vi "Variant_to_String.vi"(3 "error in (no error)":errorcluster, 5 "Variant":variant) -> (0 "error out":errorcluster, 2 "String":string)   [LabVIEW 2015]
doc: "Use this VI to change any data into a string."
panel:
  # "Creator: Branson Darnell\nEmail: bdarnell@enviroptics.com\n\nEmail me if you encounter issues with this VI."
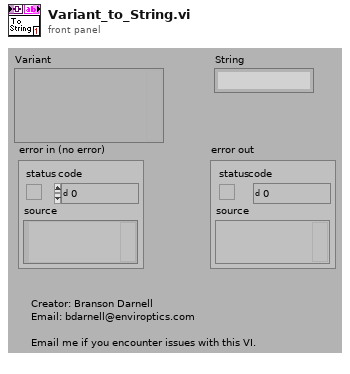
[diagram p1: front panel]
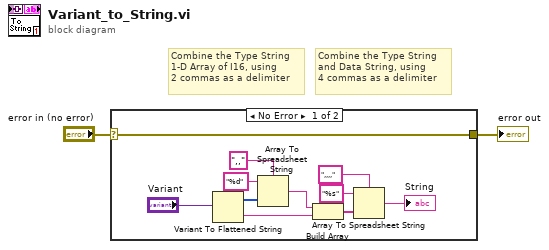
[diagram p0: block diagram]
diagram:
  # "Combine the Type String\nand Data String, using\n4 commas as a delimiter"
  # "Combine the Type String\n1-D Array of I16, using\n2 commas as a delimiter"
  n1 = case shown="No Error" "error in (no error)" {
    selector: "error in (no error)" -> [w7 w14]
    tunnel: [w7 w14] -> w1
    frame No Error {
      n2 = Variant To Flattened String(Variant="Variant") -> (data string=w10:string, 1:w9:i16[])
      n3 = Array To Spreadsheet String(delimiter (Tab)=",,", array=w9, 3:"%d" ("format string")) -> (spreadsheet string=w11:string)
      n4 = Build Array(w11, w10) -> (w12:string[])
      n5 = Array To Spreadsheet String(delimiter (Tab)=",,,,", array=w12, 3:"%s" ("format string")) -> (spreadsheet string=→"String":string)
    }
    frame Error {
    }
  }
  "error out" <- w1
